vi "path_label_dialog.vi"(5 "match patten":string, 7 "default folder path":path, 8 "error in (no error)":errorcluster, 10 "Label in":string caption="Label", 11 "Path in":path caption="Path") -> (0 "error out":errorcluster, 2 "Label out":string, 3 "Path out":path, 4 "cancelled?":bool)   [LabVIEW 2010]
panel:
  in  "cancel button":bool
  in  "ok button":bool
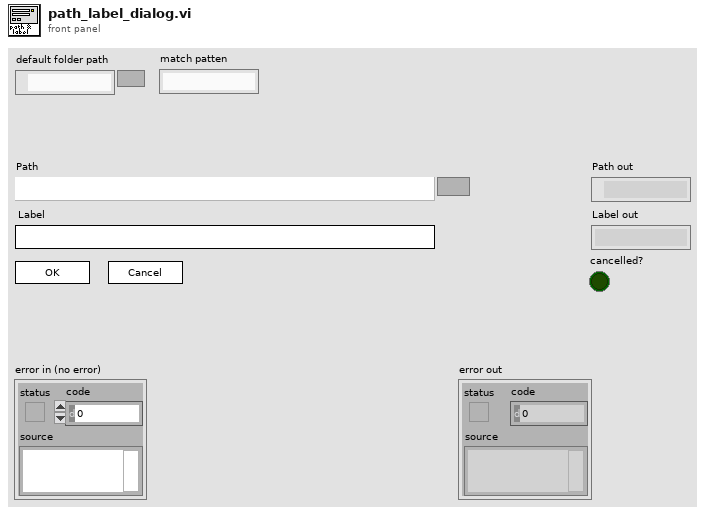
[diagram p1: front panel]
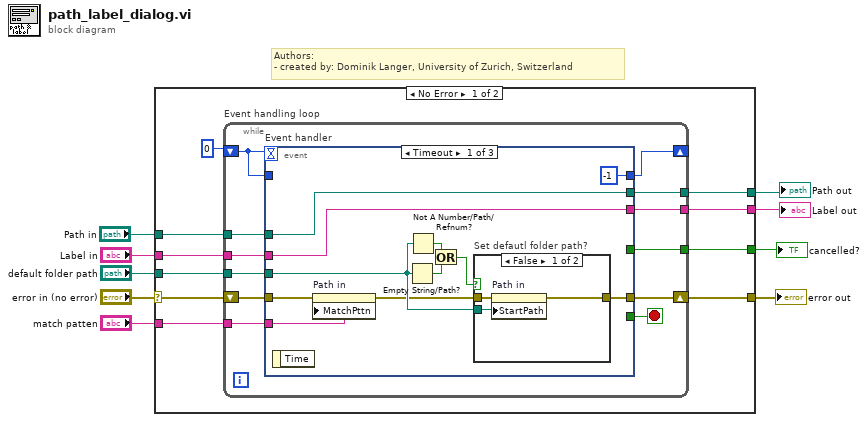
[diagram p0: block diagram]
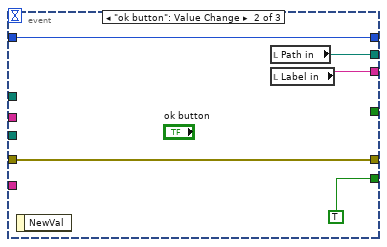
[diagram p3: hidden frame]
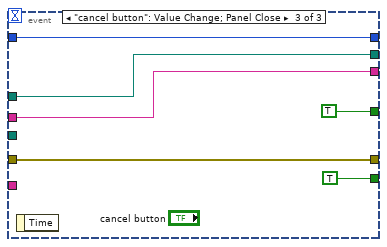
[diagram p4: hidden frame]
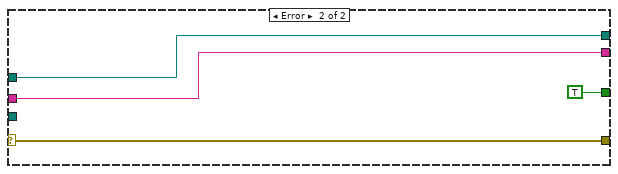
[diagram p5: hidden frame]
diagram:
  # "Authors: \n- created by: Dominik Langer, University of Zurich, Switzerland"
  n1 = case shown="No Error" "error in (no error)" {
    selector: "error in (no error)" -> [w19 w61]
    tunnel: [w18 w61] -> w8
    tunnel: "Path in" -> [w16 w60]
    tunnel: "Label in" -> [w15 w59]
    tunnel: [w14 w60] -> w5
    tunnel: [w13 w59] -> w4
    tunnel: [w12 TRUE] -> w3
    tunnel: "default folder path" -> [w11 _]
    tunnel: "match patten" -> [w10 _]
    frame No Error {
      n2 = while "Event handling loop" {
        shift-right: [w30] -> w18
        shift-left: w19 -> [w31]
        shift-right: [w28] -> _
        shift-left: 0 -> [w29]
        tunnel: w16 -> [w27]
        tunnel: w15 -> [w26]
        tunnel: [w25] -> w14
        tunnel: [w24] -> w13
        tunnel: [w22] -> w12
        tunnel: w11 -> [w21]
        tunnel: w10 -> [w20]
        stop <- w23 stop-if-true
        n3 = event "Event handler" shown="[0] Timeout" {
          selector: _ -> [_ _ _]
          dyn-events: _ -> [_ _ _]
          timeout: w29 -> [_ _ _]
          tunnel: [w39 w51 w57] -> w30
          tunnel: w31 -> [w34 w51 w57]
          tunnel: [-1 w50 w56] -> w28
          tunnel: w29 -> [_ w50 w56]
          tunnel: w27 -> [w42 _ w55]
          tunnel: w26 -> [w41 _ w54]
          tunnel: [w42 w49 w55] -> w25
          tunnel: [w41 w48 w54] -> w24
          tunnel: [_ TRUE TRUE] -> w23
          tunnel: [_ _ TRUE] -> w22
          tunnel: w21 -> [w35 _ _]
          tunnel: w20 -> [w32 _ _]
          event Timeout {
            n4 = event-data() -> ()  [unwired: 1 in, 1 out]
            n5 = property on="Path in" class="Path"(error in=w34, "MatchPttn"=w32) -> (error out=w33:errorcluster)  [unwired: 1 in, 1 out]
            n6 = Empty String/Path?(string/path=w35) -> (empty?=w36:bool)
            n7 = Not A Number/Path/Refnum?(number/path/refnum=w35) -> (NaN/Path/Refnum?=w37:bool)
            n8 = Or(x=w37, y=w36) -> (x .or. y?=w38:bool)
            n9 = case "Set defautl folder path?" shown="False" w38 {
              tunnel: w33 -> [w45 w46]
              tunnel: [w44 w46] -> w39
              tunnel: w35 -> [w43 _]
              frame False {
                n10 = property on="Path in" class="Path"(error in=w45, "StartPath"=w43) -> (error out=w44:errorcluster)  [unwired: 1 in, 1 out]
              }
              frame True {
              }
            }
          }
          event "ok button": Value Change {
            n11 = event-data() -> ()  [unwired: 1 in, 1 out]
            n12 = local read "Path in"() -> (w49:path)
            n13 = local read "Label in"() -> (w48:string)
          }
          event "cancel button": Value Change; Panel Close {
            n14 = event-data() -> ()  [unwired: 1 in, 1 out]
          }
        }
      }
    }
    frame Error {
    }
  }
  "error out" <- w8
  "Label out" <- w4
  "Path out" <- w5
  "cancelled?" <- w3
